vi "Add State Frame.vi"(8 "error in (no error)":errorcluster, 10 "element":string, 11 "CSM-Helper in":refnum<class "CSM-Helper.lvclass">) -> (0 "error out":errorcluster, 2 "Add Frame":refnum<vi>, 3 "CSM-Helper out":refnum<class "CSM-Helper.lvclass">)   [LabVIEW 2020, in "CSM-Helper.lvclass"]
uses:
  CSM-Helper.lvclass
  CSM-Helper.lvclass/CSM-Helper.ctl
  Properties/Read Case Structure Ref.vi
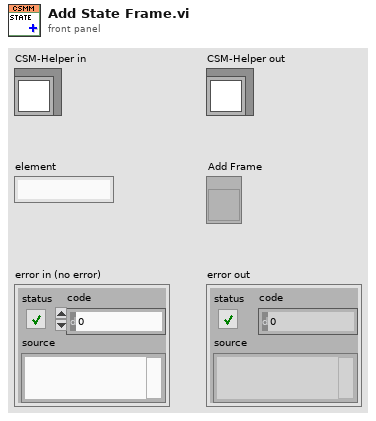
[diagram p1: front panel]
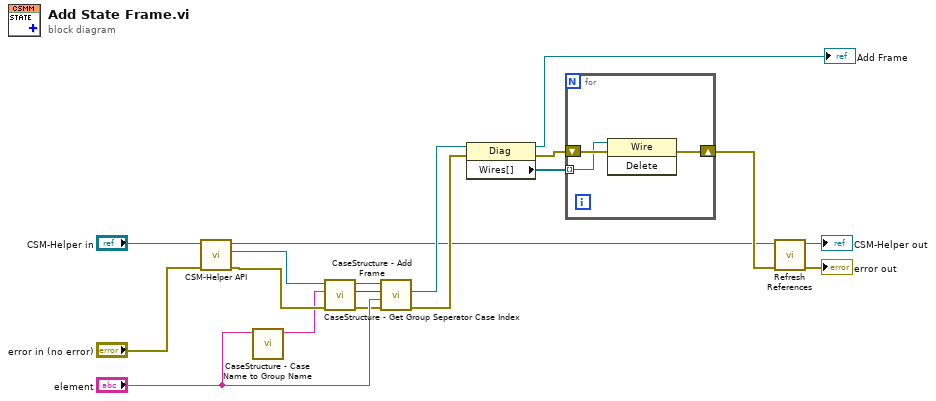
[diagram p0: block diagram]
diagram:
  n1 = call-poly "CSM-Helper API.vi"("error in (no error)"="error in (no error)", "CSM-Helper in"="CSM-Helper in") -> ("error out"=w11:errorcluster, "Case Structure"=w2:refnum<vi>, "CSM-Helper out"=w9:refnum<class "CSM-Helper.lvclass">)  [unwired: 7 in]
  n2 = call "CaseStructure - Case Name to Group Name.vi"("element"="element") -> ("String"=w6:string)  [unwired: 10 in]
  n3 = call "CaseStructure - Get Group Seperator Case Index.vi"("error in (no error)"=w11, "Group Name"=w6, "CaseStructure in"=w2) -> ("error out"=w3:errorcluster, "Numeric"=w5:i32, "CaseStructure out"=w4:refnum<vi>)  [unwired: 6 in]
  n4 = call "CaseStructure - Add Frame.vi"("error in (no error)"=w3, "Case Name"="element", "Reference Frame Index"=w5, "CaseStructure in"=w4) -> ("error out"=w14:errorcluster, "Add Frame"=w16:refnum<vi>)  [unwired: 5 in, 1 out]
  n5 = property on="Property Node" class="Diag"(reference=w16, error in=w14) -> (reference out=→"Add Frame":refnum<vi>, error out=w12:errorcluster, "Wires[]"=w13:refnum<vi>[])
  n6 = for {
    shift-right: [w21] -> w15
    shift-left: w12 -> [w20]
    tunnel: w13 -> [w19] mode=indexing
    n7 = invoke class="Wire" method="Delete"(reference=w19, error in=w20) -> (error out=w21:errorcluster)  [unwired: 1 in, 2 out]
  }
  n8 = call "Refresh References.vi"("error in (no error)"=w15, "CSM-Helper in"=w9) -> ("error out"=→"error out":errorcluster, "CSM-Helper out"=→"CSM-Helper out":refnum<class "CSM-Helper.lvclass">)  [unwired: 8 in]
